vi "Construct - File.vi"(10 "section":string, 11 "config file":path) -> (0 "Error Out":errorcluster, 3 "SQLite Database":refnum<class "SQLite Database.lvclass">)   [LabVIEW 2019, in "TSC Event Logger.lvlib" / "SQLite Database.lvclass"]
uses:
  SQLite Database.lvclass
  C:/Development/Reuse-libraries/Event Logger/Log Sinks/Log Sinks.lvclass
  Layouts/DBLayout/DBLayout.lvclass
  C:/Development/Reuse-libraries/Event Logger/Layouts/Layout.lvclass
  SQLite Database.lvclass/SQLite Database.ctl
  Log Sinks.lvclass/Log Sinks.ctl
  <vilib>/Utility/config.llb/Read Key (Path).vi
  <vilib>/Utility/config.llb/Read Key (String).vi
  <vilib>/Utility/config.llb/Read Key (Double).vi
  <vilib>/Utility/config.llb/Read Key (U32).vi
  <vilib>/Utility/config.llb/NI_LVConfig.lvlib
  Log Sinks.lvclass
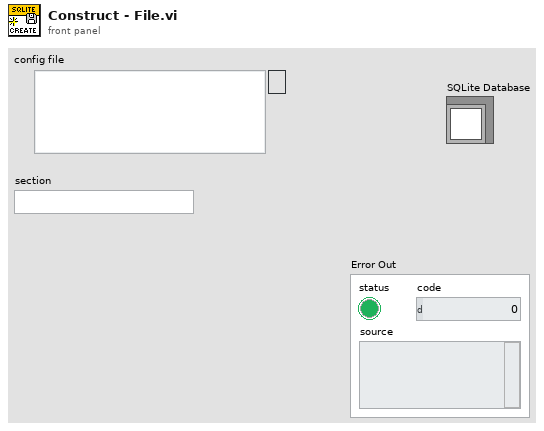
[diagram p1: front panel]
types:
  T1 = typedef "NI_LVConfig.lvlib/Config Data RefNum.ctl" = refnum<k1>
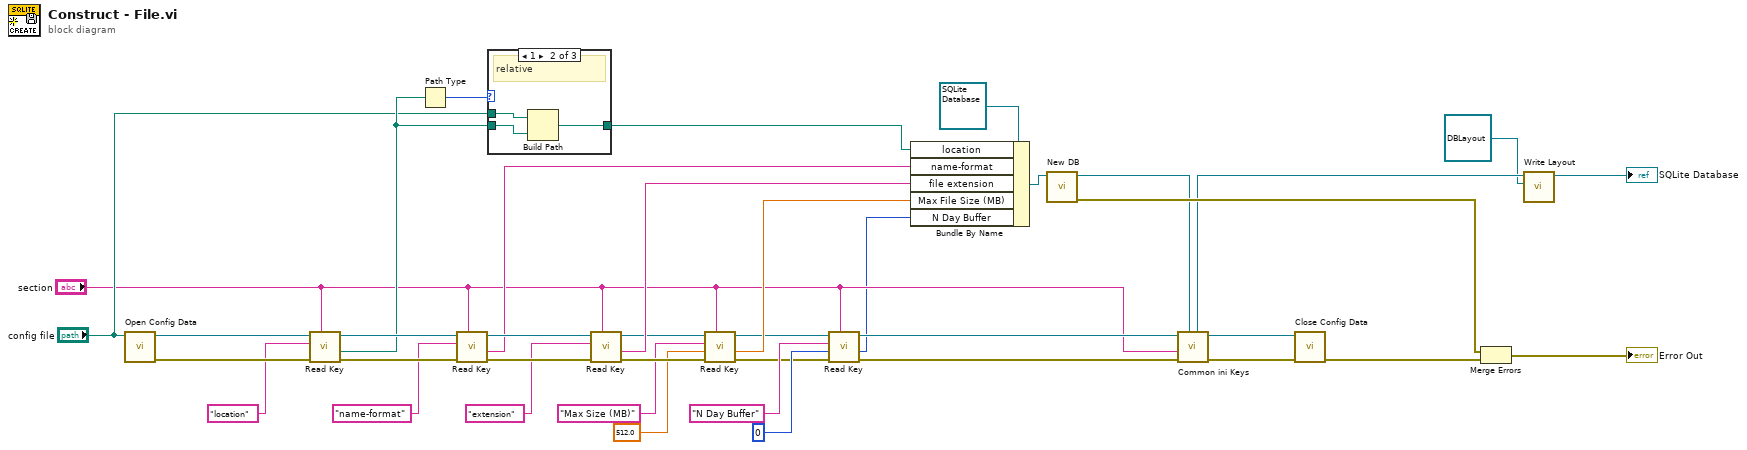
[diagram p0: block diagram]
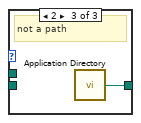
[diagram p3: hidden frame]
diagram:
  n1 = call <vilib>:"Open Config Data.vi"("configuration file path"="config file") -> ("error out"=w38:errorcluster, "refnum"=w36:T1)  [unwired: 8 in, 1 out]
  n2 = call-poly <vilib>:"Read Key.vi"("section"="section", "error in (no error)"=w38, "key"="location", "refnum"=w36) -> ("error out"=w37:errorcluster, "value"=w13:path, "refnum out"=w33:T1)  [unwired: 4 in, 1 out]
  n3 = Path Type(1:w13) -> (0:w14:i16)
  n4 = call-poly <vilib>:"Read Key.vi"("section"="section", "error in (no error)"=w37, "key"="name-format", "refnum"=w33) -> ("error out"=w34:errorcluster, "value"=w25:string, "refnum out"=w30:T1)  [unwired: 4 in, 1 out]
  n5 = case shown="1" w14 {
    tunnel: w13 -> [w40 w42 _]
    tunnel: [w40 w41 w44] -> w12
    tunnel: "config file" -> [_ w43 _]
    frame 0, Default {
      # "absolute"
    }
    frame 1 {
      # "relative"
      n6 = Build Path(base path=w43, name or relative path=w42) -> (appended path=w41:path)
    }
    frame 2 {
      # "not a path"
      n7 = call <vilib>:"Application Directory.vi"() -> ("Application Directory"=w44:path)
    }
  }
  n8 = call-poly <vilib>:"Read Key.vi"("section"="section", "error in (no error)"=w34, "key"="extension", "refnum"=w30) -> ("error out"=w31:errorcluster, "value"=w23:string, "refnum out"=w22:T1)  [unwired: 4 in, 1 out]
  n9 = call-poly <vilib>:"Read Key.vi"("section"="section", "error in (no error)"=w31, "default value"=512.0, "key"="Max Size (MB)", "refnum"=w22) -> ("error out"=w8:errorcluster, "value"=w19:dbl, "refnum out"=w7:T1)  [unwired: 3 in, 1 out]
  n10 = call-poly <vilib>:"Read Key.vi"("section"="section", "error in (no error)"=w8, "default value"=u32 0, "key"="N Day Buffer", "refnum"=w7) -> ("error out"=w6:errorcluster, "value"=w3:u32, "refnum out"=w5:T1)  [unwired: 3 in, 1 out]
  n11 = Bundle By Name(cluster=refnum<class "SQLite Database.lvclass"> refnum ("TSC Event Logger.lvlib:SQLite Database.lvclass"), "location"=w12, "name-format"=w25, "file extension"=w23, "Max File Size (MB)"=w19, "N Day Buffer"=w3) -> (w24:refnum<class "SQLite Database.lvclass">)
  n12 = call "New DB.vi"("SQLite Database in"=w24) -> ("error out"=w27:errorcluster, "SQLite Database out"=w17:refnum<class "SQLite Database.lvclass">)  [unwired: 9 in]
  n13 = call "Common ini Keys.vi"("Log Sinks in"=w17, "error in (no error)"=w6, "section"="section", "refnum in"=w5) -> ("error out"=w18:errorcluster, "refnum out"=w15:T1, "Log Sinks out"=w16:refnum<class "SQLite Database.lvclass">)  [unwired: 5 in]
  n14 = call <vilib>:"Close Config Data.vi"("error in (no error)"=w18, "refnum"=w15) -> ("error out"=w39:errorcluster)  [unwired: 8 in, 1 out]
  n15 = Merge Errors(w27, w39) -> (→"Error Out":errorcluster)
  n16 = call "Write Layout.vi"("Layout"=refnum<class "DBLayout.lvclass"> refnum ("TSC Event Logger.lvlib:DBLayout.lvclass"), "Log Sinks in"=w16) -> ("Log Sinks out"=→"SQLite Database":refnum<class "SQLite Database.lvclass">)  [unwired: 9 in]
